vi "filepath-selection-vi.vi"() -> (3 "Filepath out":T1={"Log Filepath Source"=enum."Application Relative (Auto)", "Log File Path (Manual)"=path "C:/Users/dheard/Documents/0002-labview-projects/ammonia-absorbsion-rig/data", "Log File Folder Name"="data", "log file name"="log", "Include Date in Filename"=TRUE, "Include Time in Filename"=TRUE})   [LabVIEW 2024]
uses:
  csv-file-logging/filepath-selection.ctl
panel:
  in  "Filepath Selection":T1={"Log Filepath Source"=enum."Application Relative (Auto)", "Log File Path (Manual)"=path "C:/Users/dheard/Documents/0002-labview-projects/ammonia-absorbsion-rig/data", "Log File Folder Name"="data", "log file name"="log", "Include Date in Filename"=TRUE, "Include Time in Filename"=TRUE}
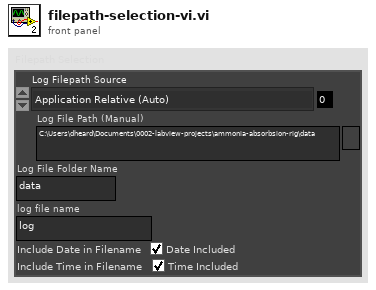
[diagram p1: front panel]
types:
  T1 = typedef "filepath-selection.ctl" = cluster{"Log Filepath Source":enum16{"Application Relative (Auto)", "VI Relative (Auto)", "Complete Path (Manual)"}, "Log File Path (Manual)":path, "Log File Folder Name":string, "log file name":string, "Include Date in Filename":bool, "Include Time in Filename":bool}
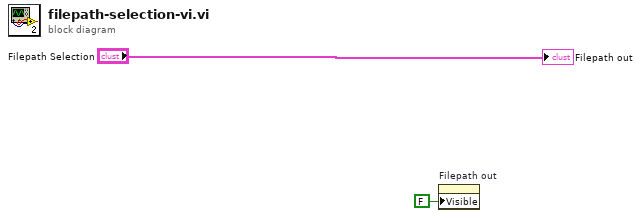
[diagram p0: block diagram]
diagram:
  n1 = property on="Filepath out" class="Clust (strict)"("Visible"=FALSE) -> ()  [unwired: 2 in, 2 out]
  "Filepath out" <- "Filepath Selection"
